vi "Fetch Core.vi"(8 "error in (no error)":errorcluster, 10 "maximum time (5s)":dbl[unit]=5000.0 caption="maximum time (5000 ms)", 11 "IVI_DMM in":refnum<class "IVI_DMM.lvclass">) -> (0 "error out":errorcluster, 2 "reading":dbl, 3 "IVI_DMM out":refnum<class "IVI_DMM.lvclass">)   [LabVIEW 2015, in "IVI_DMM.lvlib" / "IVI_DMM.lvclass"]
doc: "This VI returns the value from a previously initiated measurement.\n\nYou must first call the IviDmm Initiate VI to initiate a measurement before calling this VI.\n\nNotes:\n\n(1) After this VI executes, the Reading parameter contains an actual reading or a value indicating that an over-range condition occurred.\n\n(2) If an over-range condition occurs, the Reading parameter contains an IEEE defined NaN (Not a Number) value and the VI returns the IVIDMM_WARN_OVER_RANGE (0x3FFA2001) warning code. \n\n(3) You can test the measurement value for an over-range conditiion by calling the IviDmm Is Over-Range VI.\n\n(4) The class driver returns a simulated measurement when this VI is called and the IviDmm>>Inherent IVI Settings>>User Options>>Simulate property is set to TRUE and the IviDmm>>Inherent IVI Settings>>User Options>>Use Specific Simulation property is set to FALSE. For information on how to configure a simulated measurement, refer to the online help manual.\n\n(5) This VI does not check the instrument status. Typically, you call this VI only in a sequence of calls to other low-level driver VIs. The sequence performs one operation. You use the low-level VIs to optimize one or more aspects of interaction with the instrument. If you want to check the instrument status, call the IviDmm Error-Query VI at the conclusion of the sequence."
uses:
  IVI_DMM.lvclass
  IVI_DMM.lvclass/IVI_DMM.ctl
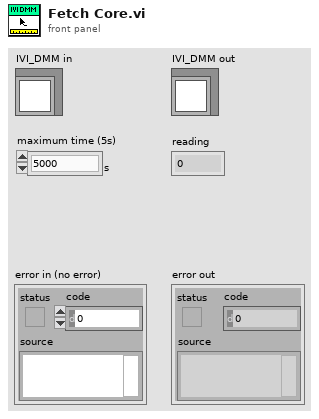
[diagram p1: front panel]
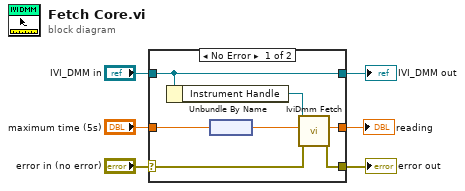
[diagram p0: block diagram]
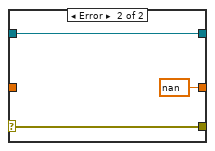
[diagram p2: hidden frame]
diagram:
  n1 = case shown="No Error" "error in (no error)" {
    selector: "error in (no error)" -> [w11 w16]
    tunnel: [w10 w16] -> w1
    tunnel: [w13 w15] -> w2
    tunnel: "IVI_DMM in" -> [w13 w15]
    tunnel: [w9 nan ("reading")] -> w4
    tunnel: "maximum time (5s)" -> [w8 _]
    frame No Error {
      n2 = Unbundle By Name(w13) -> ("Instrument Handle"=w12:refnum<k15>)
      n3 = node(w8) -> (w7:dbl)
      n4 = call <vilib>:"IviDmm Fetch.vi"("error in (no error)"=w11, "maximum time (5000 ms)"=w7, "instrument handle"=w12) -> ("error out"=w10:errorcluster, "reading"=w9:dbl)  [unwired: 5 in, 1 out]
    }
    frame Error {
    }
  }
  "error out" <- w1
  "IVI_DMM out" <- w2
  "reading" <- w4
